vi "reconnect.vi"(11 "error in (no error)":errorcluster, 13 "abort":bool) -> (4 "function return":string, 10 "serial no":string, 15 "error out":errorcluster)   [LabVIEW 2017, in "ZBOX_IS.lvlib"]
uses:
  ZBOX_IS.lvlib
panel:
  out "x > 0?":bool
  out "function return 5":string
  out "function return 4":string
  in  "milliseconds to wait":u32
  out "function return 3":string
  out "function return 2":string
  out "Numeric":i32
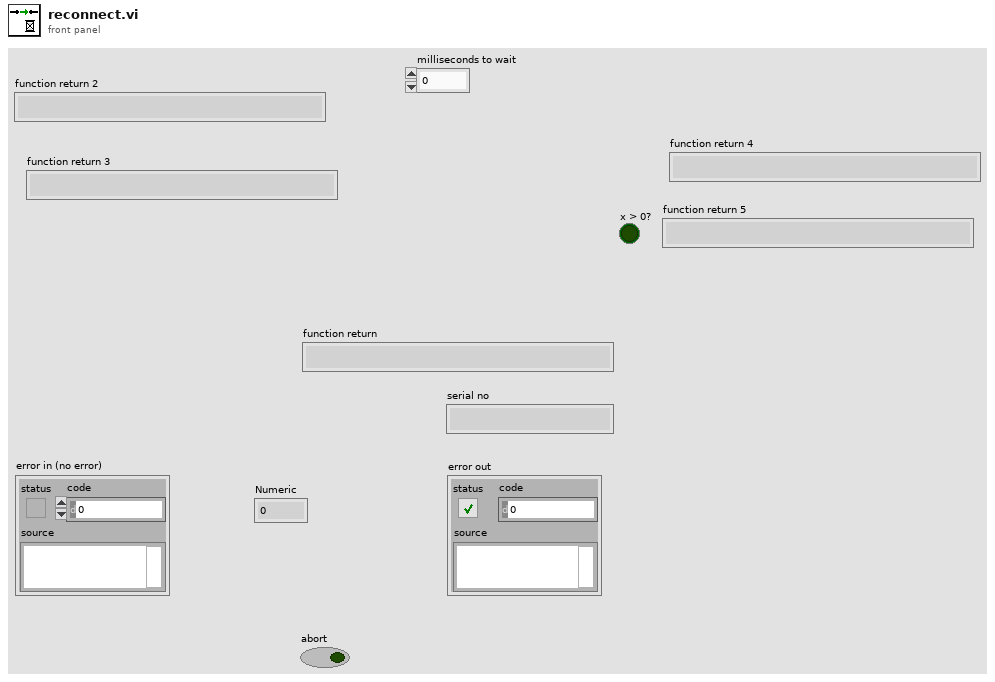
[diagram p1: front panel]
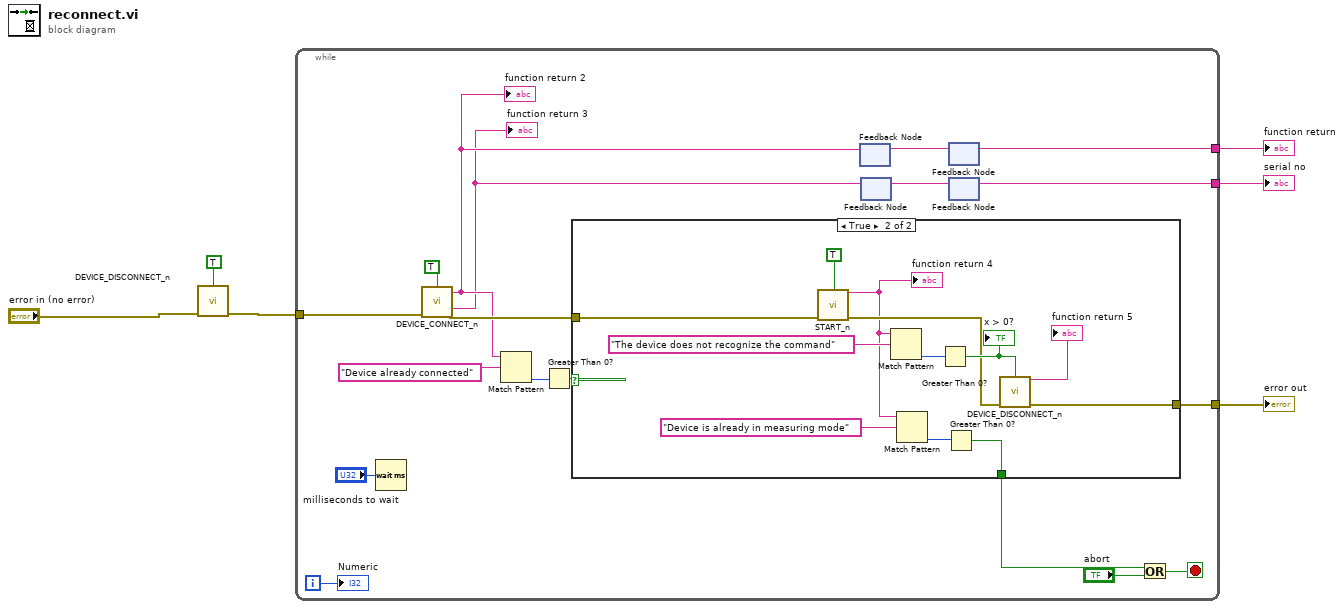
[diagram p0: block diagram]
diagram:
  n1 = call "DEVICE_DISCONNECT_n.vi"("execute"=TRUE, "error in (no error)"="error in (no error)") -> ("error out"=w4:errorcluster)  [unwired: 12 in, 1 out]
  n2 = while {
    tunnel: [w15] -> w6
    tunnel: w4 -> [w14]
    tunnel: [w10] -> w2
    tunnel: [w12] -> w1
    i -> [w17]
    stop <- w19 stop-if-true
    n3 = Wait (ms)(milliseconds to wait="milliseconds to wait") -> ()  [unwired: 1 out]
    n4 = call "DEVICE_CONNECT_n.vi"("execute"=TRUE, "error in (no error)"=w14) -> ("function return"=w8:string, "serial no"=w7:string, "error out"=w16:errorcluster)  [unwired: 10 in, 1 out]
    "function return 2" <- w8
    "function return 3" <- w7
    n5 = Match Pattern(string=w8, regular expression="Device already connected" ("substring 2")) -> (offset past match=w22:i32)  [unwired: 1 in, 3 out]
    n6 = Greater Than 0?(x=w22) -> (x > 0?=w23:bool)
    n7 = case shown="True" w23 {
      tunnel: [_ w31] -> w20
      tunnel: w16 -> [w25 w30]
      tunnel: [w25 w28] -> w15
      frame False {
      }
      frame True {
        n8 = call "START_n.vi"("execute"=TRUE, "error in (no error)"=w30) -> ("function return"=w27:string, "error out"=w29:errorcluster)  [unwired: 12 in]
        "function return 4" <- w27
        n9 = Match Pattern(string=w27, regular expression="The device does not recognize the command" ("substring 2")) -> (offset past match=w33:i32)  [unwired: 1 in, 3 out]
        n10 = Match Pattern(string=w27, regular expression="Device is already in measuring mode" ("substring 2")) -> (offset past match=w36:i32)  [unwired: 1 in, 3 out]
        n11 = Greater Than 0?(x=w33) -> (x > 0?=w32:bool)
        "x > 0?" <- w32
        n12 = Greater Than 0?(x=w36) -> (x > 0?=w31:bool)
        n13 = call "DEVICE_DISCONNECT_n.vi"("execute"=w32, "error in (no error)"=w29) -> ("function return"=→"function return 5":string, "error out"=w28:errorcluster)  [unwired: 12 in]
      }
    }
    n14 = feedback-in #1(w8) -> ()
    n15 = feedback #1() -> (w13:string)  [unwired: 1 in]
    n16 = feedback #2() -> (w11:string)  [unwired: 1 in]
    n17 = feedback-in #2(w7) -> ()
    n18 = feedback #3() -> (w12:string)  [unwired: 1 in]
    n19 = feedback-in #3(w13) -> ()
    n20 = feedback #4() -> (w10:string)  [unwired: 1 in]
    n21 = feedback-in #4(w11) -> ()
    n22 = Or(x=w20, y="abort") -> (x .or. y?=w19:bool)
    "Numeric" <- w17
  }
  "error out" <- w6
  "serial no" <- w2
  "function return" <- w1
